vi "Register Grid Click Callback.vi"(8 "error in":errorcluster, 11 "SourceGrid in":refnum<class "SourceGrid.lvclass">) -> (0 "error out":errorcluster, 3 "SourceGrid out":refnum<class "SourceGrid.lvclass">)   [LabVIEW 2023, in "SourceGrid.lvlib" / "SourceGrid.lvclass"]
uses:
  SourceGrid.lvclass
  SourceGrid.lvclass/SourceGrid.ctl
  Grid Click Callback.vi
  D:/git/Sourcegrid-LabVIEW/dll/SourceGrid.dll
  dll/SourceGrid.dll
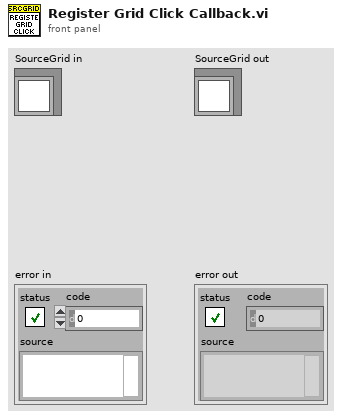
[diagram p1: front panel]
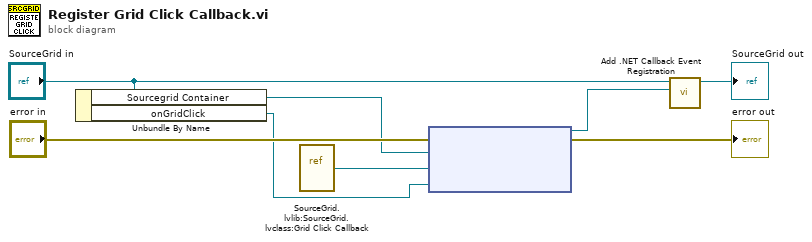
[diagram p0: block diagram]
diagram:
  n1 = Unbundle By Name("SourceGrid in") -> ("Sourcegrid Container"=w1:refnum<k24>, "onGridClick"=w5:refnum<user-event>)
  n2 = vi-ref "SourceGrid.lvlib:SourceGrid.lvclass:Grid Click Callback.vi"() -> ("vi reference"=w4:refnum<vi>)
  n3 = node("error in", w1, w4, w5) -> (w2:refnum<k27>, →"error out":errorcluster)  [unwired: 1 in]
  n4 = call "Add .NET Callback Event Registration.vi"("Event Callback Refnum"=w2, "SourceGrid in"="SourceGrid in") -> ("SourceGrid out"=→"SourceGrid out":refnum<class "SourceGrid.lvclass">)  [unwired: 9 in]
